vi "Teleop.vi"(10 "Match Info":T2={"Autonomous Elapsed Seconds"=0.0, "TeleOp Elapsed Seconds"=0.0, "Disabled Elapsed Seconds"=0.0, "Visited Autonomous"=FALSE, "Visited TeleOp"=FALSE, "Visited Disabled"=FALSE, "Autonomous Settings"={"Autonomous Style"=enum."Independent", "VI Refnum"=refnum}}, 11 "Call Context":T3) -> ()   [LabVIEW 2014]
doc: "This VI is called for each TeleOp packet received from the DS where the robot is not disabled. It is often used to read from the joysticks and update I/O or to update setpoints for timed control loops. It should complete and return within 20 milliseconds or it may miss DS packets."
uses:
  <vilib>/Rock Robotics/WPI/DriverStation/WPI_DriverStationDerivedRobotMode.ctl
  <vilib>/Rock Robotics/WPI/DriverStation/WPI_DriverStationMatch Info.ctl
  <vilib>/Rock Robotics/WPI/Solenoid/WPI_SolenoidValue.ctl
  <vilib>/Rock Robotics/Network Tables/SD Read Boolean.vi
  <vilib>/Rock Robotics/Network Tables/SD Read Number.vi
  <vilib>/Rock Robotics/WPI/Joystick/WPI_JoystickGetSetRefNum.vi
  <vilib>/Rock Robotics/Network Tables/SD Write Boolean Array.vi
  <vilib>/Rock Robotics/Network Tables/SD Write Numeric Array.vi
  <vilib>/Rock Robotics/WPI/RobotDrive/WPI_RobotDriveGetSetRefNum.vi
  <vilib>/Rock Robotics/WPI/RobotDrive/WPI_RobotDriveMecanumDrive_Cartesian.vi
  <vilib>/Rock Robotics/Network Tables/SD Write Number.vi
  <vilib>/Rock Robotics/WPI/Solenoid/WPI_SolenoidSetEnum.vi
  <vilib>/addons/control/pid/NI_PID_pid.lvlib
  <vilib>/addons/control/pid/pid.llb/PID (DBL).vi
  <vilib>/Rock Robotics/WPI/Ultrasonic/WPI_SonarSRF04DigitalGetRange.vi
  <vilib>/Rock Robotics/WPI/Ultrasonic/WPI_SonarSRF04DigitalRefNum Registry Get.vi
panel:
  out "Distance":dbl
  out "Arm Power":dbl
  out "UpperLimit":bool
  out "LowerLimit":bool
  out "Initialize Header":bool=TRUE
  out "Header":dbl
  out "PID Output":dbl format="%.2f"
  out "Gyro Angle":dbl
  in  "STRAIGHT PID":T1={"proportional gain (Kc)"=0.02, "integral time (Ti, min)"=0.05, "derivative time (Td, min)"=0.0} {"derivative time (Td, min)" format="%.3f"; "integral time (Ti, min)" format="%.3f"; "proportional gain (Kc)" format="%.3f"}
  out "X Threshold":dbl
  out "Y Threshold":dbl
  out "R Threshold":dbl
  out "X Original":dbl
  out "Y Original":dbl
  out "R Original":dbl
  out "Sample Slider 0":dbl(slide) scale=0.0..5.0
  out "Sample Boolean 1":bool
  out "Sample Boolean 0":bool
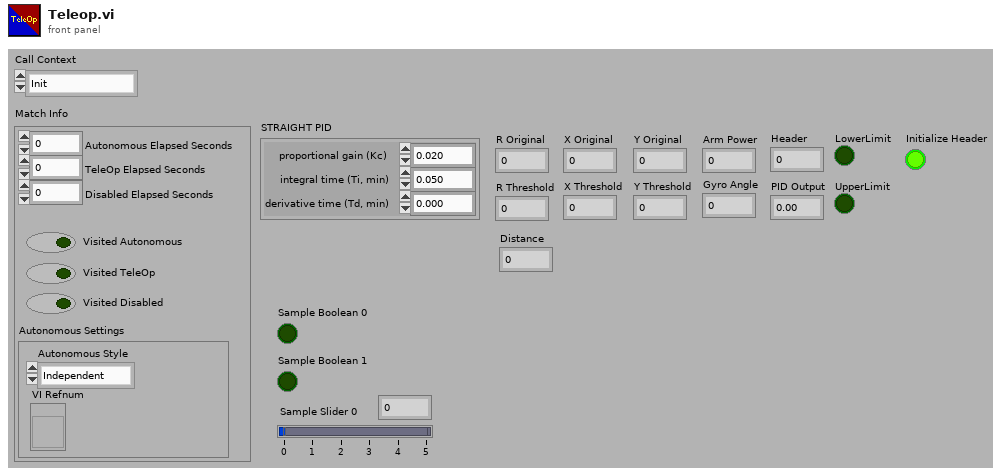
[diagram p1: front panel]
types:
  T1 = cluster{"proportional gain (Kc)":dbl, "integral time (Ti, min)":dbl, "derivative time (Td, min)":dbl}
  T2 = typedef "WPI_DriverStationMatch Info.ctl" = cluster{"Autonomous Elapsed Seconds":dbl, "TeleOp Elapsed Seconds":dbl, "Disabled Elapsed Seconds":dbl, "Visited Autonomous":bool, "Visited TeleOp":bool, "Visited Disabled":bool, "Autonomous Settings":cluster{"Autonomous Style":enum16{"Iterative", "Independent"}, "VI Refnum":refnum<vi>}}
  T3 = typedef "WPI_DriverStationDerivedRobotMode.ctl" = enum16{"Init", "Execute", "Stop"}
  T4 = typedef "WPI_SolenoidValue.ctl" = enum16{"Off", "On", "Forward", "Reverse"}
  T5 = typedef "WPI_JoystickDevRef.ctl" = cluster{"Device":T6}
  T6 = typedef "WPI_JoystickDeviceEnum.ctl" = enum16{"USB 0", "USB 1", "USB 2", "USB 3", "USB 4", "USB 5"}
  T7 = typedef "WPI_DigitalInputDevRef.ctl" = cluster{"DevStatus":errorcluster, "DIO Channel":T8, "Controller":T9}
  T8 = typedef "FPGA_DIOChannel.ctl" = enum8{"DIO 0", "DIO 1", "DIO 2", "DIO 3", "DIO 4", "DIO 5", "DIO 6", "DIO 7", "DIO 8", "DIO 9", "DIO MXP 0", "DIO MXP 1", "DIO MXP 2", "DIO MXP 3", "DIO MXP 4", "DIO MXP 5", "DIO MXP 6", "DIO MXP 7", "DIO MXP 8", "DIO MXP 9", "DIO MXP 10", "DIO MXP 11", "DIO MXP 12", "DIO MXP 13", "DIO MXP 14", "DIO MXP 15", "Invalid"}
  T9 = typedef "FPGA_TypedefDigitalModule.ctl" = enum16{"Controller 1"}
  T10 = typedef "WPI_GyroDevRef.ctl" = cluster{"DevStatus":errorcluster, "Analog Module":T11, "Analog Channel":T12, "Offset":dbl, "Gain (VoltsPerDegree/Second)":dbl}
  T11 = typedef "FPGA_TypedefAnalogModule.ctl" = enum16{"Controller 1"}
  T12 = typedef "FPGA_AIChannel.ctl" = enum8{"AI 0", "AI 1", "AI 2", "AI 3", "AI MXP 0", "AI MXP 1", "AI MXP 2", "AI MXP 3", "Invalid"}
  T13 = typedef "WPI_UltrasonicDeviceRef.ctl" = cluster{"DevStatus":errorcluster, "Ping Digital Controller":T9, "Echo Digital Controller":T9, "Ping Channel":T8, "Echo Channel":T8, "CntIndex":T14}
  T14 = typedef "FPGA_CounterCtrSystemIndex.ctl" = enum8{"Ctr 0", "Ctr 1", "Ctr 2", "Ctr 3", "Ctr 4", "Ctr 5", "Ctr 6", "Ctr 7", "Invalid"}
  T15 = typedef "WPI_SolenoidDevRef.ctl" = cluster{"DevStatus":errorcluster, "Pneumatics Control Module":u8, "Forward Solenoid Channel":T16, "Reverse Solenoid Channel":T16}
  T16 = typedef "WPI_SolenoidChannel.ctl" = enum8{"Solenoid 0", "Solenoid 1", "Solenoid 2", "Solenoid 3", "Solenoid 4", "Solenoid 5", "Solenoid 6", "Solenoid 7", "Invalid"}
  T17 = typedef "WPI_MotorControlDeviceRef.ctl" = cluster{"DeviceStatus":errorcluster, "Type":T18, "PWM":cluster{"Controller":T9, "PWM Channel":T19, "DeadBand":T20}, "CAN":cluster{"Device Number":u8, "Control Mode":T21, "Semaphore":T22, "Max Vout":dbl, "TalonSRX Control Mode":T23}, "Invert":bool, "TransformRef":T24, "InvTransformRef":T24}
  T18 = typedef "WPI_MotorControlType.ctl" = enum16{"PWM", "CAN", "CANTalonSRX"}
  T19 = typedef "FPGA_DIOPWMChannel.ctl" = enum8{"PWM 0", "PWM 1", "PWM 2", "PWM 3", "PWM 4", "PWM 5", "PWM 6", "PWM 7", "PWM 8", "PWM 9", "PWM MXP 0", "PWM MXP 1", "PWM MXP 2", "PWM MXP 3", "PWM MXP 4", "PWM MXP 5", "PWM MXP 6", "PWM MXP 7", "PWM MXP 8", "PWM MXP 9", "Invalid"}
  T20 = typedef "WPI_PWMDeadband.ctl" = cluster{"Name":string, "maxPositivePwm":i32, "minPositivePwm":i32, "centerPwm":i32, "maxNegativePwm":i32, "minNegativePwm":i32, "angularRange":u16}
  T21 = typedef "WPI_CANJaguar_ControlMode.ctl" = enum8{"Percent VBus", "Current", "Speed", "Position", "Voltage"}
  T22 = typedef "Semaphore RefNum" = refnum<k1>
  T23 = typedef "WPI_CANTalonSRX_APIControlMode.ctl" = enum8{"Percent VBus", "Speed", "Position", "Slave", "Unchanged / Invalid"}
  T24 = typedef "WPI_PWMTransform_ConPane.ctl" = refnum<vi>
  T25 = typedef "WPI_RobotDriveDevRef.ctl" = cluster{"DevStatus":errorcluster, "Motors[]":T17[], "Square Inputs":bool, "Max Output":dbl}
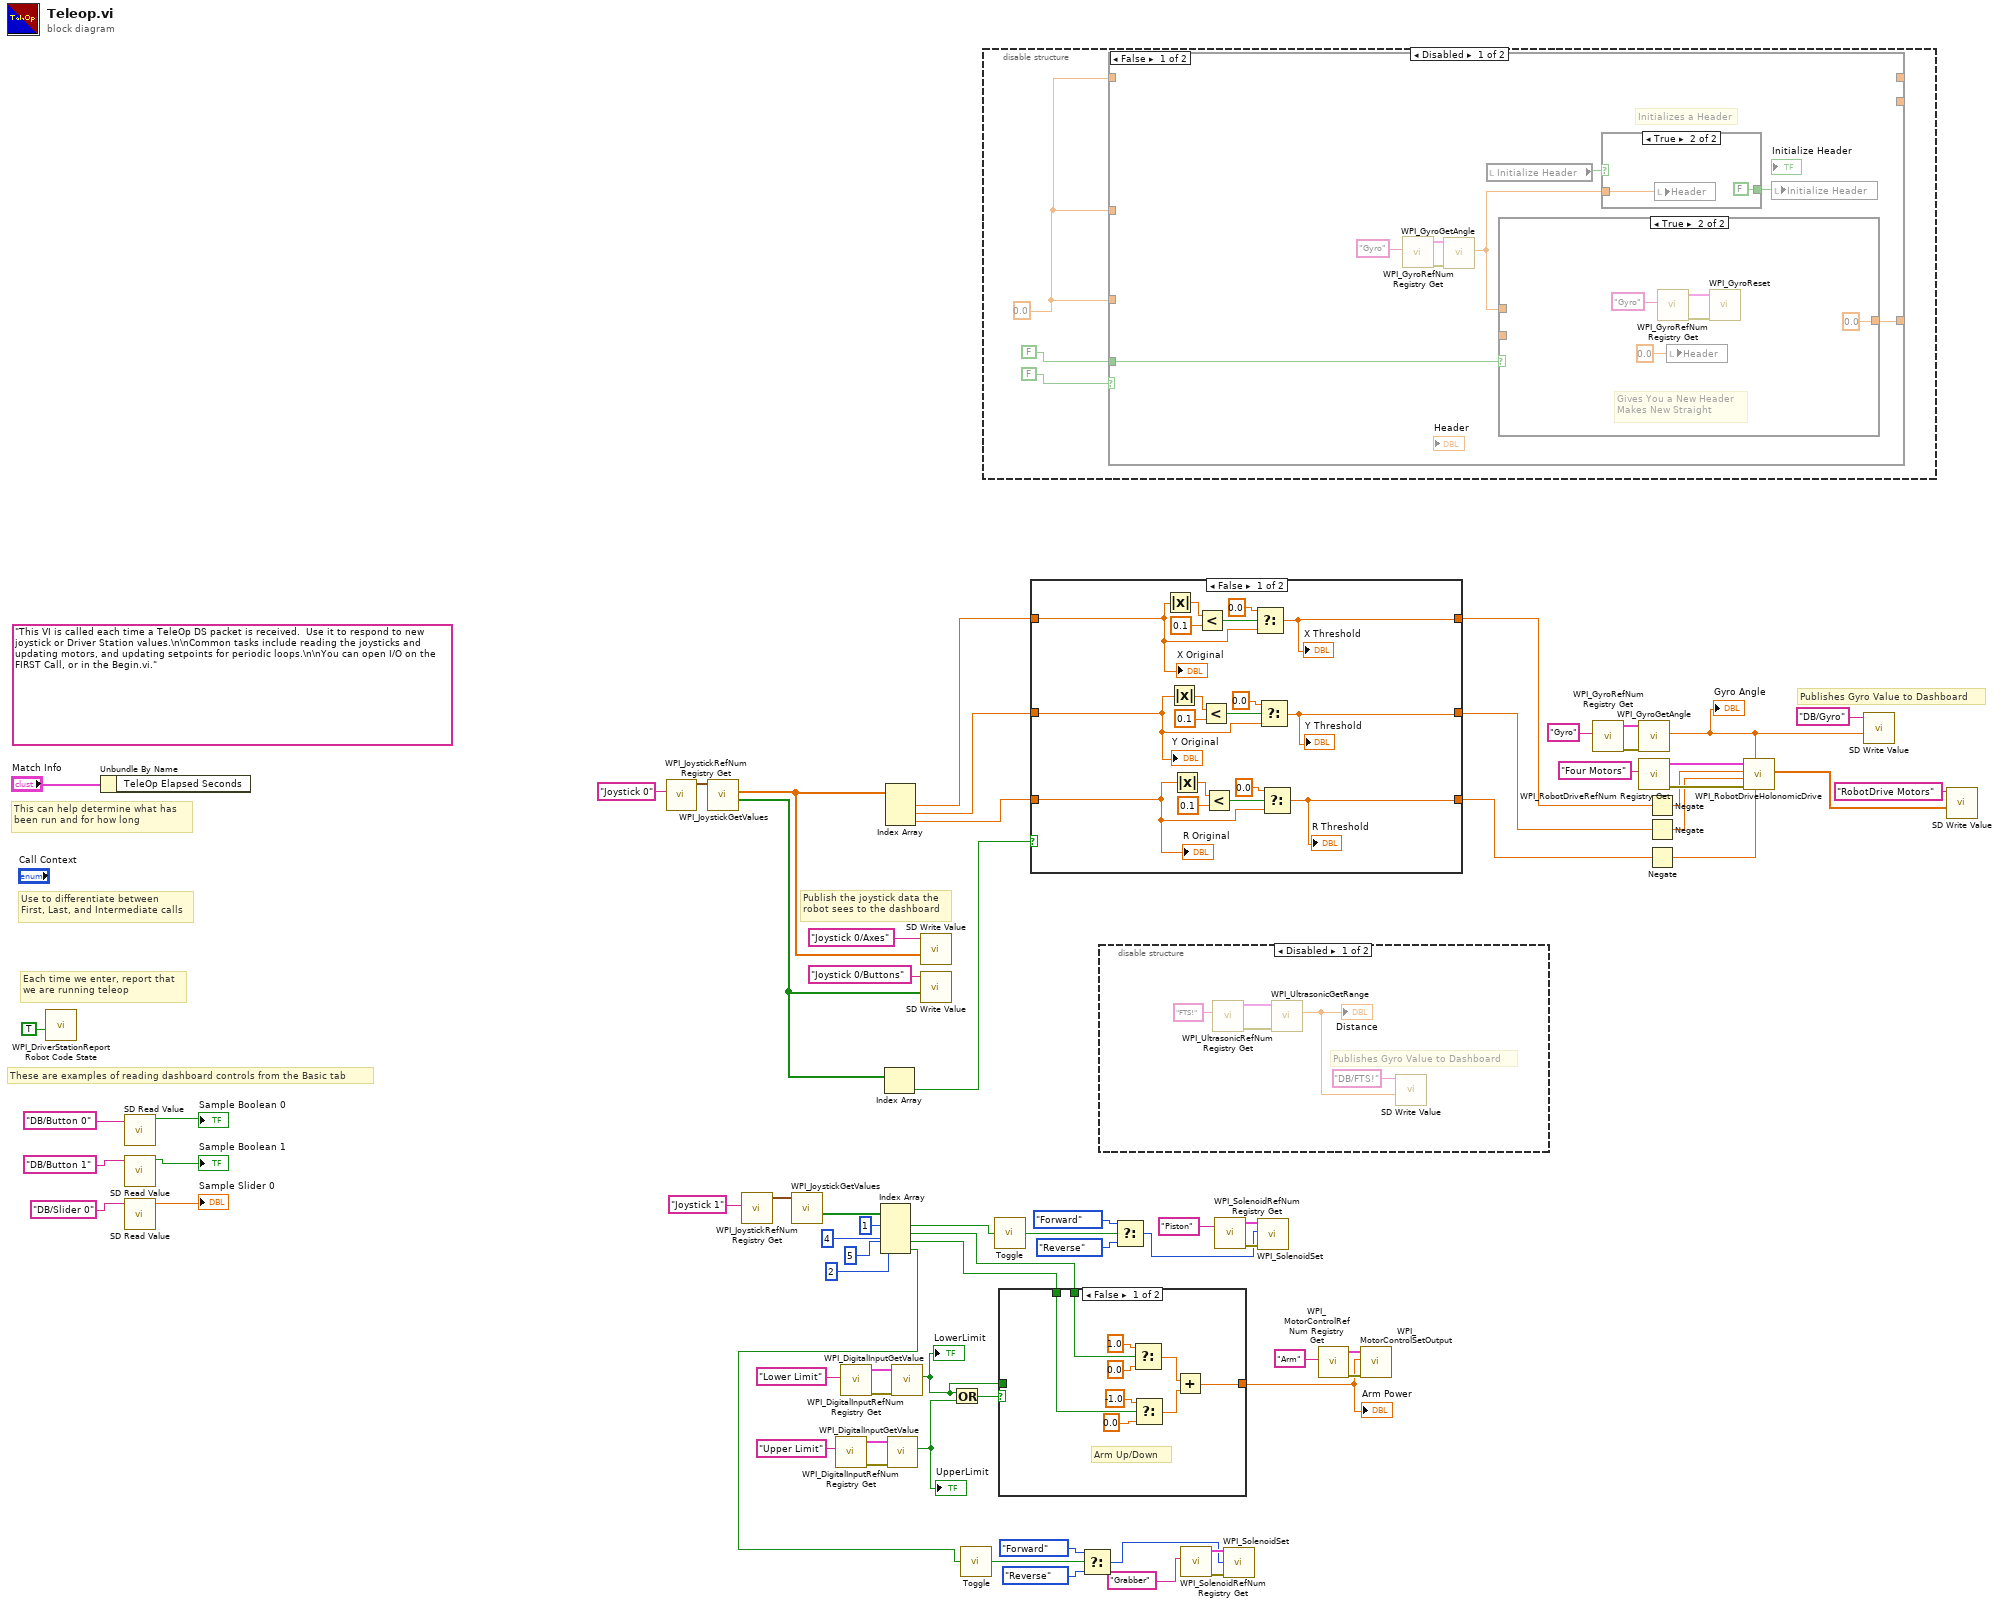
[diagram p0: block diagram]
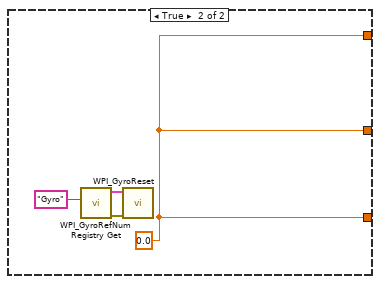
[diagram p3: hidden frame]
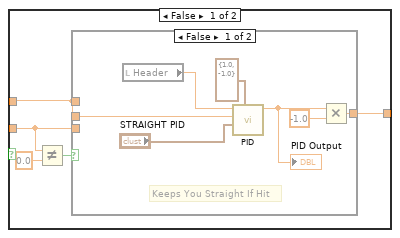
[diagram p4: hidden frame]
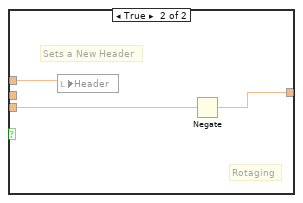
[diagram p5: hidden frame]
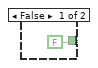
[diagram p6: hidden frame]
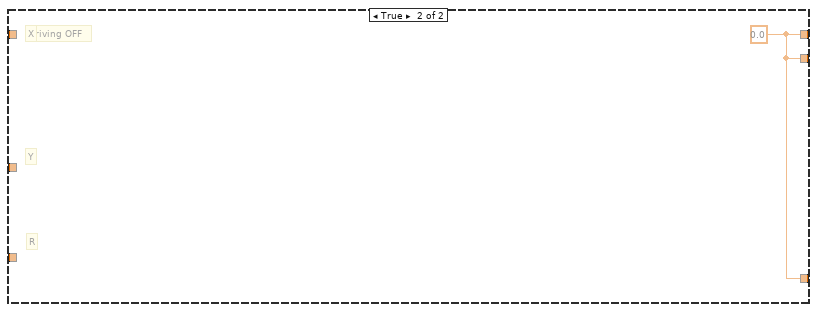
[diagram p7: hidden frame]
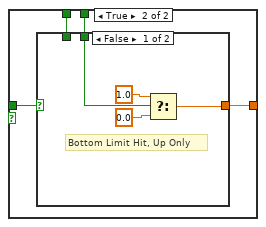
[diagram p9: hidden frame]
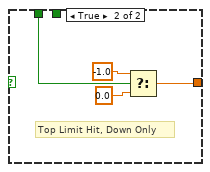
[diagram p10: hidden frame]
diagram:
  (unwired) "This VI is called each time a TeleOp DS packet is received.  Use it to respond to new joystick or Driver Station values.\n\nCommon tasks include reading the joysticks and updating motors, and updating setpoints for periodic loops.\n\nYou can open I/O on the FIRST Call, or in the Begin.vi."
  # "Publishes Gyro Value to Dashboard"
  # "Publish the joystick data the\nrobot sees to the dashboard"
  # "These are examples of reading dashboard controls from the Basic tab"
  # "Each time we enter, report that\nwe are running teleop"
  # "Use to differentiate between\nFirst, Last, and Intermediate calls"
  # "This can help determine what has\nbeen run and for how long"
  n1 = call <vilib>:"WPI_DriverStationReport Robot Code State.vi"("TeleOp"=TRUE ("Autonomous")) -> ()  [unwired: 10 in, 1 out]
  n2 = Unbundle By Name("Match Info") -> ()  [unwired: 1 out]
  n3 = call-poly <vilib>:"SD Read Value.vi"("Name"="DB/Button 0" ("refnum name")) -> ("Boolean"=→"Sample Boolean 0":bool)  [unwired: 8 in, 2 out]
  n4 = call-poly <vilib>:"SD Read Value.vi"("Name"="DB/Button 1" ("refnum name")) -> ("Boolean"=→"Sample Boolean 1":bool)  [unwired: 8 in, 2 out]
  n5 = call-poly <vilib>:"SD Read Value.vi"("Name"="DB/Slider 0" ("refnum name")) -> ("Numeric"=→"Sample Slider 0":dbl)  [unwired: 8 in, 2 out]
  n6 = call <vilib>:"WPI_JoystickRefNum Registry Get.vi"("refnum name"="Joystick 0") -> ("JoystickDevRef"=w54:T5)  [unwired: 1 in, 9 out]
  n7 = call <vilib>:"WPI_JoystickGetValues.vi"("JoystickDevRef"=w54) -> ("Buttons"=w44:bool[], "Axes"=w49:dbl[])  [unwired: 6 in, 3 out]
  n8 = call <vilib>:"WPI_JoystickRefNum Registry Get.vi"("refnum name"="Joystick 1") -> ("JoystickDevRef"=w58:T5)  [unwired: 1 in, 9 out]
  n9 = call <vilib>:"WPI_JoystickGetValues.vi"("JoystickDevRef"=w58) -> ("Buttons"=w59:bool[])  [unwired: 6 in, 4 out]
  n10 = call <vilib>:"WPI_DigitalInputRefNum Registry Get.vi"("refnum name"="Upper Limit") -> ("error out"=w39:errorcluster, "DigitalInputDevRef"=w40:T7)  [unwired: 9 in]
  n11 = call <vilib>:"WPI_DigitalInputRefNum Registry Get.vi"("refnum name"="Lower Limit") -> ("error out"=w42:errorcluster, "DigitalInputDevRef"=w41:T7)  [unwired: 9 in]
  n12 = Index Array(array=w59, index #1=1 ("index"), index #2=4 ("index"), index #3=5 ("index"), index #4=2 ("index")) -> (element #1=w12:bool, element #2=w11:bool, element #3=w10:bool, element #4=w9:bool)
  n13 = Index Array(array=w44) -> (element=w13:bool)  [unwired: 1 in]
  n14 = Index Array(array=w49) -> (element #1=w20:dbl, element #2=w18:dbl, element #3=w14:dbl)  [unwired: 3 in]
  n15 = call <vilib>:"WPI_DigitalInputGetValue.vi"("error in (no error)"=w39, "DigitalInputDevRef"=w40) -> ("Value"=w33:bool)  [unwired: 7 in, 2 out]
  "UpperLimit" <- w33
  n16 = call <vilib>:"WPI_DigitalInputGetValue.vi"("error in (no error)"=w42, "DigitalInputDevRef"=w41) -> ("Value"=w34:bool)  [unwired: 7 in, 2 out]
  "LowerLimit" <- w34
  n17 = call-poly <vilib>:"SD Write Value.vi"("Numeric Array"=w49, "Name"="Joystick 0/Axes") -> ()  [unwired: 8 in, 2 out]
  n18 = call-poly <vilib>:"SD Write Value.vi"("Boolean Array"=w44, "Name"="Joystick 0/Buttons") -> ()  [unwired: 8 in, 2 out]
  n19 = Or(x=w34, y=w33) -> (x .or. y?=w21:bool)
  n20 = call "Toggle.vi"("Input"=w9) -> ("Output"=w27:bool)
  n21 = disable-structure shown="Disabled" {
    frame Disabled {
      w73 = 0.0 ("upper limit")
      n22 = case shown="False" FALSE ("Output") {
        tunnel: [w83 w107] -> _
        tunnel: w73 -> [_ _]
        tunnel: w73 -> [_ _]
        tunnel: FALSE -> [w80 _]
        tunnel: [_ w107] -> _
        tunnel: w73 -> [_ _]
        tunnel: [_ w107] -> _
        frame False {
          # "Initializes a Header"
          n23 = call <vilib>:"WPI_GyroRefNum Registry Get.vi"("refnum name"="Gyro") -> ("error out"=w76:errorcluster, "GyroDevRef"=w78:T10)  [unwired: 9 in]
          n24 = call <vilib>:"WPI_GyroGetAngle.vi"("error in (no error)"=w76, "GyroDevRef"=w78) -> ("Angle"=w77:dbl)  [unwired: 6 in, 3 out]
          n25 = local read "Initialize Header"() -> (w82:bool)
          n26 = case shown="True" w80 {
            tunnel: [w88 0.0] -> w83
            tunnel: _ -> [w85 _]
            tunnel: w77 -> [w84 _]
            frame False {
              n27 = Not Equal?(x=w85, y=0.0) -> (x != y?=w86:bool)
              n28 = case shown="False" w86 {
                tunnel: [w94 w96] -> w88
                tunnel: w84 -> [w95 _]
                tunnel: w84 -> [_ w98]
                tunnel: w85 -> [_ w97]
                frame False {
                  # "Keeps You Straight If Hit"
                  n29 = local read "Header"() -> (w91:dbl)
                  n30 = call-poly <vilib>:"PID.vi"("output range"=cluster{"output high":dbl, "output low":dbl} {"output high"=1.0, "output low"=-1.0}, "PID gains"="STRAIGHT PID", "process variable"=w95, "setpoint"=w91) -> ("output"=w90:dbl)  [unwired: 6 in, 1 out]
                  "PID Output" <- w90
                  n31 = Multiply(x=w90, y=-1.0) -> (x*y=w94:dbl)
                }
                frame True {
                  # "Sets a New Header"
                  # "Rotaging"
                  n32 = local write "Header"(w98) -> ()
                  n33 = Negate(x=w97) -> (-x=w96:dbl)
                }
              }
            }
            frame True {
              # "Gives You a New Header\nMakes New Straight"
              n34 = call <vilib>:"WPI_GyroRefNum Registry Get.vi"("refnum name"="Gyro") -> ("error out"=w102:errorcluster, "GyroDevRef"=w101:T10)  [unwired: 9 in]
              n35 = local write "Header"(0.0 ("Header 2")) -> ()
              n36 = call <vilib>:"WPI_GyroReset.vi"("error in (no error)"=w102, "GyroDevRef"=w101) -> ()  [unwired: 8 in, 2 out]
            }
          }
          n37 = case shown="True" w82 {
            tunnel: w77 -> [_ w106]
            tunnel: [FALSE FALSE] -> w81
            frame False {
            }
            frame True {
              n38 = local write "Header"(w106) -> ()
            }
          }
          n39 = local write "Initialize Header"(w81) -> ()
        }
        frame True {
          w107 = 0.0 ("upper limit")
          # "R"
          # "Y"
          # "X"
          # "Driving OFF"
        }
      }
    }
    frame Enabled {
    }
  }
  n40 = call "Toggle.vi"("Input"=w12) -> ("Output"=w28:bool)
  n41 = case shown="False" w21 {
    tunnel: w11 -> [w112 w118]
    tunnel: w10 -> [w111 w119]
    tunnel: [w108 w117] -> w29
    tunnel: w34 -> [_ w120]
    frame False {
      # "Arm Up/Down"
      n42 = Select(t=1.0 ("Output"), s=w112, f=0.0) -> (s? t:f=w109:dbl)
      n43 = Select(t=-1.0 ("Output"), s=w111, f=0.0) -> (s? t:f=w110:dbl)
      n44 = Add(x=w109, y=w110) -> (x+y=w108:dbl)
    }
    frame True {
      n45 = case shown="False" w120 {
        tunnel: w119 -> [_ w128]
        tunnel: w118 -> [w124 _]
        tunnel: [w121 w125] -> w117
        frame False {
          # "Bottom Limit Hit, Up Only"
          n46 = Select(t=1.0, s=w124, f=0.0) -> (s? t:f=w121:dbl)
        }
        frame True {
          # "Top Limit Hit, Down Only"
          n47 = Select(t=-1.0, s=w128, f=0.0) -> (s? t:f=w125:dbl)
        }
      }
    }
  }
  "Arm Power" <- w29
  n48 = case shown="False" w13 {
    tunnel: [w141 w150] -> w2
    tunnel: w20 -> [w142 _]
    tunnel: w18 -> [w136 _]
    tunnel: [w135 w150] -> w19
    tunnel: w14 -> [w130 _]
    tunnel: [w129 w150] -> w15
    frame False {
      n49 = Absolute Value(x=w142) -> (abs(x)=w146:dbl)
      n50 = Absolute Value(x=w136) -> (abs(x)=w140:dbl)
      n51 = Absolute Value(x=w130) -> (abs(x)=w131:dbl)
      n52 = Less?(x=w146, y=0.1) -> (x < y?=w144:bool)
      n53 = Less?(x=w140, y=0.1) -> (x < y?=w138:bool)
      n54 = Less?(x=w131, y=0.1) -> (x < y?=w133:bool)
      n55 = Select(t=0.0, s=w144, f=w142) -> (s? t:f=w141:dbl)
      "X Threshold" <- w141
      n56 = Select(t=0.0, s=w138, f=w136) -> (s? t:f=w135:dbl)
      "Y Threshold" <- w135
      n57 = Select(t=0.0, s=w133, f=w130) -> (s? t:f=w129:dbl)
      "R Threshold" <- w129
      "X Original" <- w142
      "Y Original" <- w136
      "R Original" <- w130
    }
    frame True {
      w150 = 0.0 ("upper limit")
      n58 = call <vilib>:"WPI_GyroRefNum Registry Get.vi"("refnum name"="Gyro") -> ("error out"=w147:errorcluster, "GyroDevRef"=w148:T10)  [unwired: 9 in]
      n59 = call <vilib>:"WPI_GyroReset.vi"("error in (no error)"=w147, "GyroDevRef"=w148) -> ()  [unwired: 8 in, 2 out]
    }
  }
  n60 = Select(t=WPI_SolenoidValue."Forward" ("Value"), s=w27, f=WPI_SolenoidValue."Reverse" ("Value")) -> (s? t:f=w22:T4)
  n61 = disable-structure shown="Disabled" {
    frame Disabled {
      # "Publishes Gyro Value to Dashboard"
      n62 = call-poly <vilib>:"WPI_UltrasonicRefNum Registry Get.vi"("refnum name"="FTS!") -> ("error out"=w155:errorcluster, "SonarSRF04DevRef"=w154:T13)  [unwired: 9 in]
      n63 = call-poly <vilib>:"WPI_UltrasonicGetRange.vi"("error in (no error)"=w155, "SonarSRF04DevRef"=w154) -> ("Distance"=w151:dbl)  [unwired: 7 in, 2 out]
      "Distance" <- w151
      n64 = call-poly <vilib>:"SD Write Value.vi"("Numeric"=w151, "Name"="DB/FTS!") -> ()  [unwired: 8 in, 2 out]
    }
    frame Enabled {
    }
  }
  n65 = Select(t=WPI_SolenoidValue."Forward" ("Value"), s=w28, f=WPI_SolenoidValue."Reverse" ("Value")) -> (s? t:f=w30:T4)
  n66 = call <vilib>:"WPI_SolenoidRefNum Registry Get.vi"("refnum name"="Grabber") -> ("error out"=w24:errorcluster, "SolenoidDevRef"=w23:T15)  [unwired: 9 in]
  n67 = call <vilib>:"WPI_SolenoidRefNum Registry Get.vi"("refnum name"="Piston") -> ("error out"=w62:errorcluster, "SolenoidDevRef"=w63:T15)  [unwired: 9 in]
  n68 = call-poly <vilib>:"WPI_SolenoidSet.vi"("error in (no error)"=w24, "Value"=w22, "SolenoidDevRef"=w23) -> ()  [unwired: 7 in, 2 out]
  n69 = call-poly <vilib>:"WPI_SolenoidSet.vi"("error in (no error)"=w62, "Value"=w30, "SolenoidDevRef"=w63) -> ()  [unwired: 7 in, 2 out]
  n70 = call <vilib>:"WPI_MotorControlRefNum Registry Get.vi"("refnum name"="Arm") -> ("error out"=w36:errorcluster, "MotorControlDevRef"=w37:T17)  [unwired: 9 in]
  n71 = call <vilib>:"WPI_MotorControlSetOutput.vi"("error in (no error)"=w36, "Output"=w29, "MotorControlDevRef"=w37) -> ()  [unwired: 6 in, 3 out]
  n72 = call <vilib>:"WPI_GyroRefNum Registry Get.vi"("refnum name"="Gyro") -> ("error out"=w45:errorcluster, "GyroDevRef"=w47:T10)  [unwired: 9 in]
  n73 = call <vilib>:"WPI_GyroGetAngle.vi"("error in (no error)"=w45, "GyroDevRef"=w47) -> ("Angle"=w31:dbl)  [unwired: 6 in, 3 out]
  "Gyro Angle" <- w31
  n74 = call <vilib>:"WPI_RobotDriveRefNum Registry Get.vi"("refnum name"="Four Motors") -> ("error out"=w51:errorcluster, "RobotDriveDevRef"=w50:T25)  [unwired: 9 in]
  n75 = Negate(x=w2) -> (-x=w32:dbl)
  n76 = Negate(x=w19) -> (-x=w17:dbl)
  n77 = Negate(x=w15) -> (-x=w16:dbl)
  n78 = call-poly <vilib>:"WPI_RobotDriveHolonomicDrive.vi"("Rotation"=w16, "Gyro Angle"=w31, "error in (no error)"=w51, "Y"=w17, "X"=w32, "RobotDriveDevRef"=w50) -> ("Motor Values"=w3:dbl[])  [unwired: 3 in, 2 out]
  n79 = call-poly <vilib>:"SD Write Value.vi"("Numeric"=w31, "Name"="DB/Gyro") -> ()  [unwired: 8 in, 2 out]
  n80 = call-poly <vilib>:"SD Write Value.vi"("Numeric Array"=w3, "Name"="RobotDrive Motors") -> ()  [unwired: 8 in, 2 out]
